vi "Timer Double to Picture.vi"(11 "Time (sec)":dbl) -> (2 "Time":string, 3 "new picture":picture)   [LabVIEW 2021]
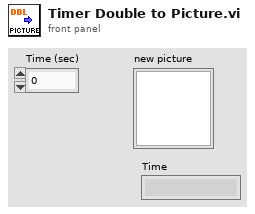
[diagram p1: front panel]
types:
  T1 = cluster{"Font Name:":string, "Size":i16, "Strikeout?":bool, "Italic?":bool, "Underline?":bool, "Outline?":bool, "Shadow?":bool, "Bold?":bool}
  T2 = enum16{"User-specified Font", "Application Font", "System Font", "Dialog Font"}
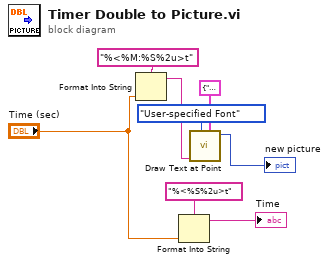
[diagram p0: block diagram]
diagram:
  n1 = Format Into String(format string="%<%M:%S%2u>t", "Time (sec)") -> (resulting string=w5:string)  [unwired: 2 in, 1 out]
  n2 = Format Into String(format string="%<%S%2u>t", "Time (sec)") -> (resulting string=→"Time":string)  [unwired: 2 in, 1 out]
  n3 = call <vilib>:"Draw Text at Point.vi"("[user-specified font]"=T1 {"Font Name:"="Verdana", "Size"=200, "Strikeout?"=FALSE, "Italic?"=FALSE, "Underline?"=FALSE, "Outline?"=FALSE, "Shadow?"=FALSE, "Bold?"=TRUE}, "desired font(Application)"=T2."User-specified Font", "text"=w5) -> ("new picture"=→"new picture":picture)  [unwired: 7 in, 1 out]
